vi "CSMLS - Add Exit State(s) with Loop Check.vi"(0 "Exiting States":string="//Exit Sub-Modules\nData: Cleanup\nExit", 5 "States Queue":string="Data: Acquisite\nDAQ: Continuous Check >> 0.331641 -><loop>\nDAQ: Stop\r\nDAQ: Close\r\nUI: Refresh Buttons -><end>") -> (6 "Remaining States":string="Data: Acquisite\r\nDAQ: Stop\r\nDAQ: Close\r\nUI: Refresh Buttons -><end>\n//Exit Sub-Modules\nData: Cleanup\nExit", 8 "<loop> Found":bool)   [LabVIEW 2017, in "CSM Loop Support.lvlib"]
doc: "Checks for loop tags upon exit. Since this VI is easily forgotten to be called, a call has been added for the \"Macro: Exit\" state in the Parse State Queue++ VI. Therefore, this VI has been removed from the Functions palette.\n\n-- <b>Controls</b> --\n- <b>States Queue</b>: Connect the entire state queue to this input.\n- <b>Exiting States</b>: States required for exiting.\n\n-- <b>Indicators</b> --\n- <b>Remaining States</b>: Processed message queue.\n- <b><loop> Found</b>: `<loop>` tag found."
uses:
  CSM Loop Support.lvlib
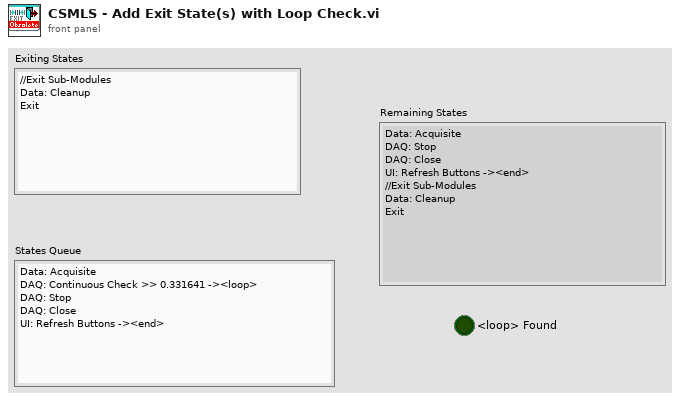
[diagram p1: front panel]
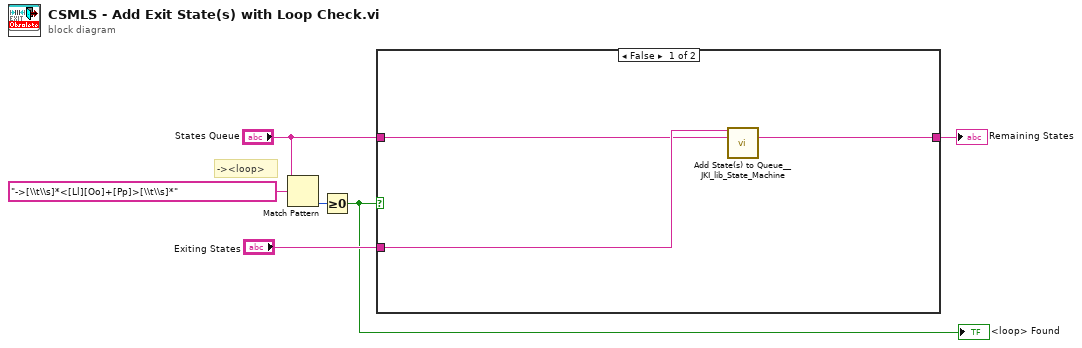
[diagram p0: block diagram]
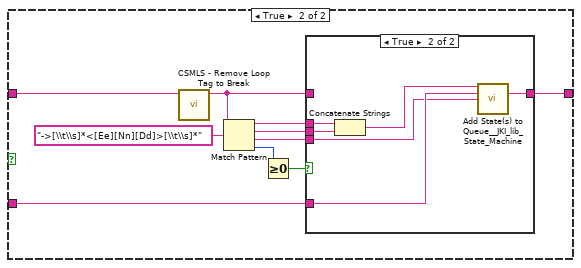
[diagram p2: hidden frame]
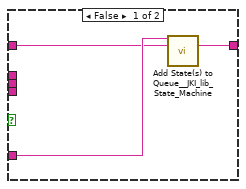
[diagram p3: hidden frame]
diagram:
  # "-><loop>"
  n1 = Match Pattern(string="States Queue", regular expression="->[\\t\\s]*<[Ll][Oo]+[Pp]>[\\t\\s]*") -> (offset past match=w5:i32)  [unwired: 1 in, 3 out]
  n2 = Greater Or Equal To 0?(x=w5) -> (x >= 0?=w1:bool)
  "<loop> Found" <- w1
  n3 = case shown="False" w1 {
    tunnel: [w9 w10] -> w3
    tunnel: "Exiting States" -> [w8 w11]
    tunnel: "States Queue" -> [w7 w19]
    frame False {
      n4 = call <vilib>:"Add State(s) to Queue__JKI_lib_State_Machine.vi"("State(s) in Front (\"\")"=w8, "State(s) in (\"\")"=w7) -> ("States Out"=w9:string)  [unwired: 13 in]
    }
    frame True {
      n5 = call "CSMLS - Remove Loop Tag to Break.vi"("States Queue"=w19) -> ("Remaining States"=w12:string)  [unwired: 10 in]
      n6 = Match Pattern(string=w12, regular expression="->[\\t\\s]*<[Ee][Nn][Dd]>[\\t\\s]*") -> (before substring=w16:string, match substring=w17:string, after substring=w18:string, offset past match=w14:i32)  [unwired: 1 in]
      n7 = Greater Or Equal To 0?(x=w14) -> (x >= 0?=w15:bool)
      n8 = case shown="True" w15 {
        tunnel: [w20 w26] -> w10
        tunnel: w12 -> [w21 _]
        tunnel: w16 -> [_ w28]
        tunnel: w17 -> [_ w27]
        tunnel: w18 -> [_ w23]
        tunnel: w11 -> [w22 w24]
        frame False {
          n9 = call <vilib>:"Add State(s) to Queue__JKI_lib_State_Machine.vi"("State(s) in Front (\"\")"=w22, "State(s) in (\"\")"=w21) -> ("States Out"=w20:string)  [unwired: 13 in]
        }
        frame True {
          n10 = Concatenate Strings(w28, w27) -> (w25:string)
          n11 = call <vilib>:"Add State(s) to Queue__JKI_lib_State_Machine.vi"("State(s) in Front (\"\")"=w25, "State(s) in (\"\")"=w24, "State(s) at Back (\"\")"=w23) -> ("States Out"=w26:string)  [unwired: 12 in]
        }
      }
    }
  }
  "Remaining States" <- w3
